vi "Master_Control.vi"(8 "error in (no error)":errorcluster, 10 "FPGA VI Reference In":refnum<k20>) -> (0 "error out":errorcluster, 2 "FPGA VI Reference Out":refnum<k20>)   [LabVIEW 2017]
doc: "The control loop on the cRIO.\nContains the state machine that sets actuations by states. The actuations vary depending on the runtype class used, set from the tab control on the Host Front Panel. Although each variation of the state has similar properties.\nContains an emergency check, watchdog pet/kick, distance approximator.\nThe runtypes are as follows:\nFullRun - pod is configured to perform a vacuum run through the tube at full speed\nSystemsCheck - manual control over all actuations is provided, including a short motor pulse feature\nService - motor is running and manual control over the pod's position is provided\nThe states are as follows:\nIdle - pod is not in motion, and is in a safe state\nReady - all subsystems are actuated and the command to send pod into launch is enabled\nPushing - pod is in motion and accelerating\nCoasting - pod is neither accelerating nor braking\nBraking - pod is braking and coming to a stop\nFault - the emergency check registered a fault and all outputs are disabled\nShutdown - the GlobalStop variable is set to true, stopping all loops running on the cRIO\nBlank - a template for easily creating new states as needed"
uses:
  TypeDef_ControlState.ctl
  RunTypesLibrary/FullRunClass/FullRun.lvclass
  C:/Users/Trevor/Documents/GitHub/SpaceXComp/Master/Control/RunTypesLibrary/RunTypeClass/RunType.lvclass
  TypeDef_DigitalOuts.ctl
  TypeDef_LoopPeriods.ctl
  <vilib>/Platform/TimedLoop/XDataNode/timing_clust.ctl
  <vilib>/Platform/TimedLoop/XDataNode/nitl_modes.ctl
  <vilib>/Platform/TimedLoop/XDataNode/wakeup.ctl
  DAQ/Master_DataControl.ctl
  DAQ/TypeDef_cRIOData.ctl
  IMU/TypeDef_IMUData.ctl
  CAN/TypeDef_BMSData.ctl
  CAN/TypeDef_BMS_Status.ctl
  CAN/MotorController/fixedMotorData.ctl
  CAN/MotorController/MotorStatus.ctl
  RunTypesLibrary/RunTypeList.ctl
  RunTypesLibrary/SystemsCheckClass/SystemsCheck.lvclass
  <vilib>/Platform/TimedLoop/XDataNode/loadnilvce.vi
  <vilib>/platform/TimedLoop/XDataNode/XDataNode.xnode
  RunTypesLibrary/RunTypeClass/RunType.lvclass
  EmergencyCheck/CheckData/CheckData.lvclass
  <vilib>/Platform/TimedLoop/XDataNode/XDNodeRunTimeDep.lvlib
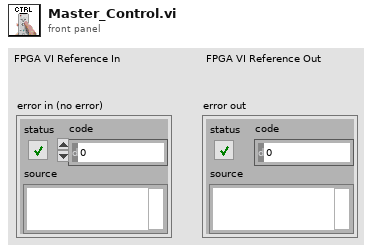
[diagram p1: front panel]
types:
  T1 = typedef "TypeDef_DigitalOuts.ctl" = cluster{"Pod Power":bool, "Dump Valve":bool, "Brakes":bool, "Clamp":bool, "Pump":bool, "Ignition":bool, "DO6":bool, "DO7":bool, "HighSide":bool, "Precharge":bool, "LowSide":bool, "DO3":bool, "DO4":bool, "DO5":bool, "DO62":bool, "DO72":bool}
  T2 = typedef "TypeDef_ControlState.ctl" = enum16{"Systems Check", "Idle", "Ready", "Pushing", "Coast", "Braking", "Fault", "Shutdown", "Service", "Precharge", "Blank"}
  T3 = typedef "TypeDef_LoopPeriods.ctl" = cluster{"Control Period":i64, "DAQ Period":u32, "IMU Period":u32, "CAN Period":i64, "Nav Period":u32}
  T4 = typedef "XDNodeRunTimeDep.lvlib/timing_clust.ctl" = cluster{"Expected End [f-1]":u64, "Actual End [f-1]":u64, "Finished Late? [f-1]":bool, "Expected End [i-1]":u64, "Actual End [i-1]":u64, "Finished Late? [i-1]":bool, "Expected Start [i]":u64, "Actual Start [i]":u64, "Expected Start [f]":u64, "Actual Start [f]":u64, "Source Name":string, "Structure Name":string, "Period":i64, "Deadline":i64, "Offset":i64, "Start":i64, "Priority":i32, "Timeout":i32, "Mode":T5, "Wakeup Reason":T6, "Error":errorcluster, "Source Type":string, "Secondary Source Type":string, "Global End Time":u64, "Global Start Time":u64, "Frame Duration":u64, "Iteration Duration":u64, "Assigned CPU":i32, "I/O Scan Engine Mode":u32}
  T5 = typedef "XDNodeRunTimeDep.lvlib/nitl_modes.ctl" = enum32{"No Change", "Process missed periods, maintain original phase", "Discard missed periods, maintain original phase", "Process missed periods, ignore original phase", "Discard missed periods, ignore original phase"}
  T6 = typedef "XDNodeRunTimeDep.lvlib/wakeup.ctl" = enum32{"Normal", "Aborted", "Asynchronous wakeup", "Timing source error", "Timed loop error", "Timeout"}
  T7 = typedef "RunTypeList.ctl" = enum16{"Full Run", "Systems Check", "Service"}
  T8 = typedef "Master_DataControl.ctl" = cluster{"cRIO Data":T9, "IMU Data":T10, "BMS Data":T11, "Motor Data":T13}
  T9 = typedef "TypeDef_cRIOData.ctl" = cluster{"Time (ms)":dbl, "24V Battery (V)":dbl, "LowV Current (A)":dbl, "Fiducial Sensor (V)":dbl, "PV Pressure (psig)":dbl, "Flow Sensor (V)":dbl, "Temp Fairing (F)":dbl, "Temp Reservoir (F)":dbl, "HallEffect Right (in)":dbl, "HallEffect Left (in)":dbl, "PT Tank (psig)":dbl, "PT Clamp Right (psig)":dbl, "PT Clamp Left (psig)":dbl, "PT Brake (psig)":dbl, "PT Cooling (psig)":dbl, "Displacement (ft)":dbl, "Velocity (ft/s)":dbl}
  T10 = typedef "TypeDef_IMUData.ctl" = cluster{"x acceleration (g)":dbl, "Pressure (psia)":dbl, "Temperature (F)":dbl}
  T11 = typedef "TypeDef_BMSData.ctl" = cluster{"Max Cell Voltage (V)":dbl, "Max Cell ID":dbl, "Min Cell Voltage (V)":dbl, "Min Cell ID":dbl, "State of Charge (%)":dbl, "Average Voltage (V)":dbl, "Voltage Delta (V)":dbl, "Pack Current (A)":dbl, "Pack Voltage (V)":dbl, "Max Resistance (Ohm)":dbl, "Min Resistance (Ohm)":dbl, "Average Resistance (Ohm)":dbl, "Delta Resistance (Ohm)":dbl, "Highest Temperature(F)":dbl, "BmsStatus":T12}
  T12 = typedef "TypeDef_BMS_Status.ctl" = cluster{"isFault":bool, "isolationMonitoring":bool}
  T13 = typedef "fixedMotorData.ctl" = cluster{"Velo (RPM)":dbl, "MotorTemp(F)":dbl, "CtrlTemp(F)":dbl, "DcLinkVolt(V)":dbl, "ErrorCode":dbl, "motorStatus":T14, "isAlive":bool, "motorControllerState":u16}
  T14 = typedef "MotorStatus.ctl" = cluster{"isReady":bool, "isOn":bool, "isOperEn":bool, "isFault":bool, "isVoltEn":bool, "targetReached":bool, "isWarning":bool}
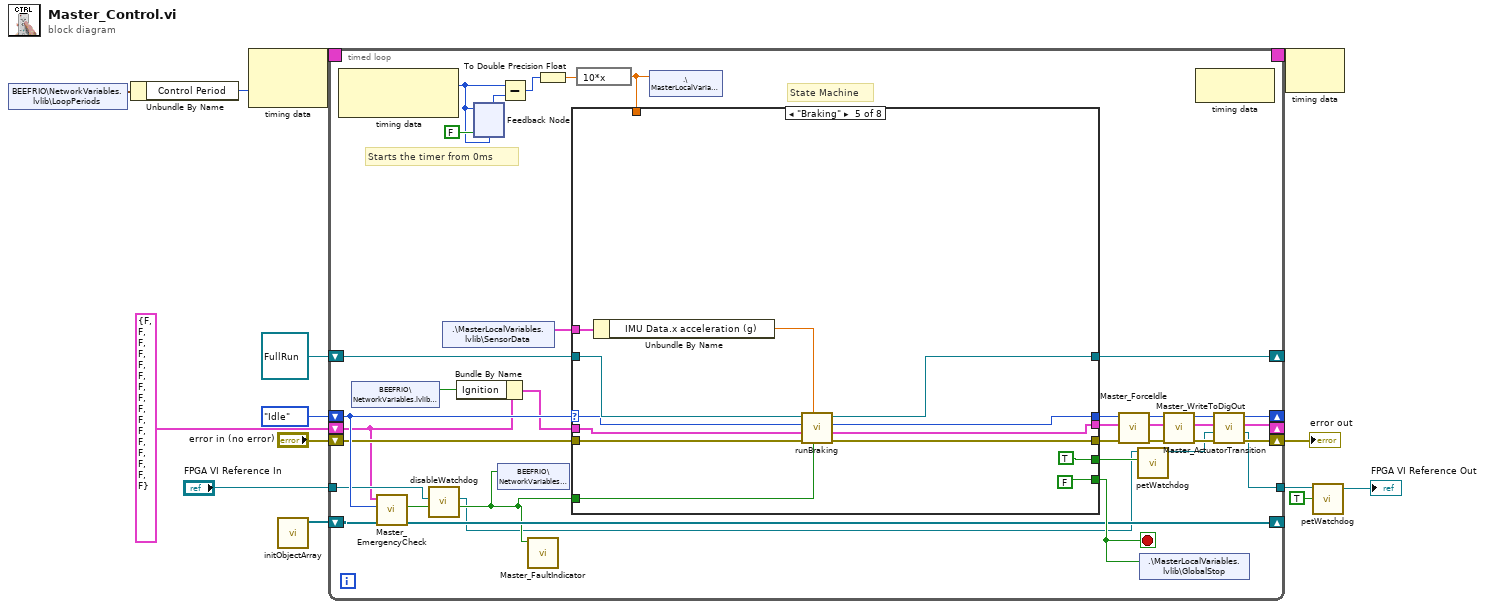
[diagram p0: block diagram]
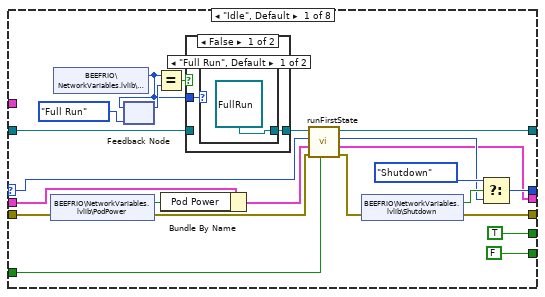
[diagram p2: hidden frame]
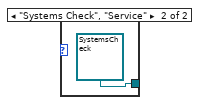
[diagram p3: hidden frame]
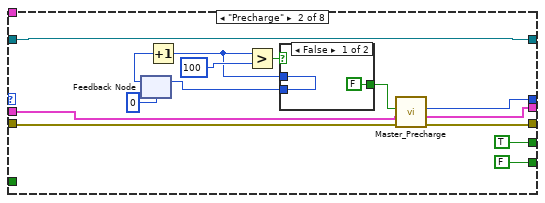
[diagram p5: hidden frame]
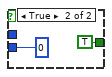
[diagram p6: hidden frame]
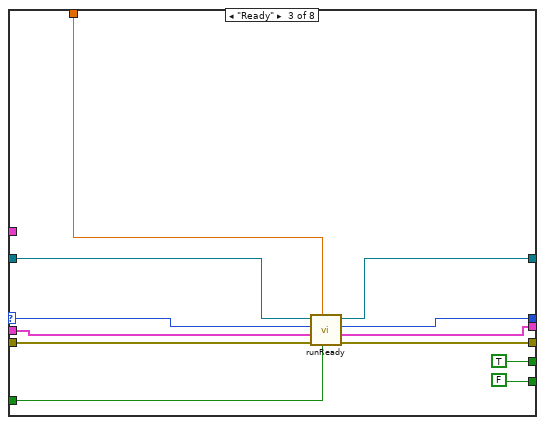
[diagram p7: hidden frame]
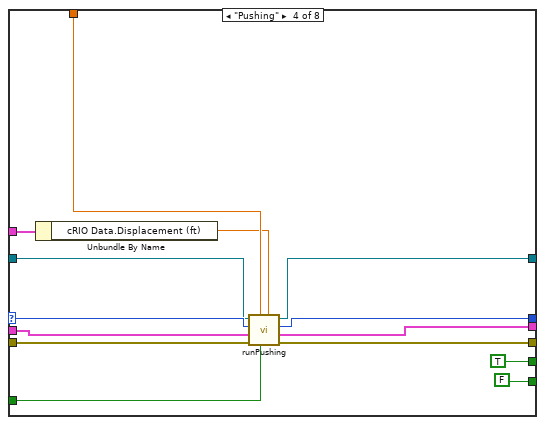
[diagram p8: hidden frame]
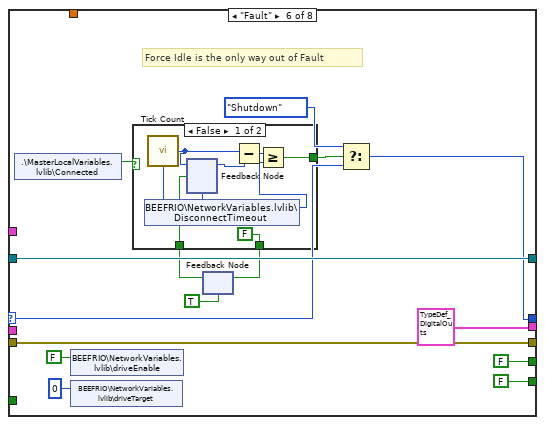
[diagram p9: hidden frame]
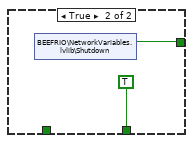
[diagram p10: hidden frame]
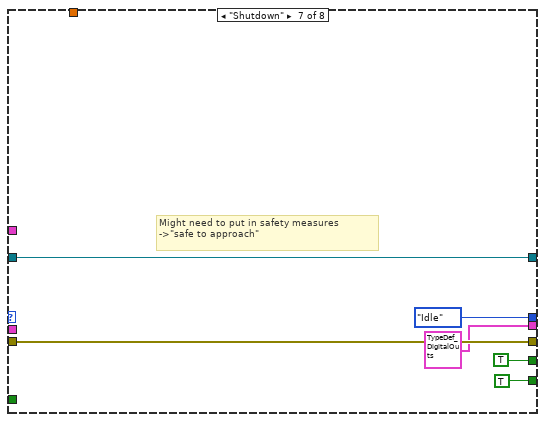
[diagram p11: hidden frame]
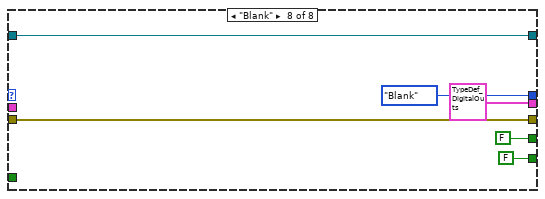
[diagram p12: hidden frame]
diagram:
  n1 = shared-variable "BEEFRIO\\NetworkVariables.lvlib\\LoopPeriods"() -> (w10:T3)  [unwired: 1 in, 1 out]
  n2 = Unbundle By Name(w10) -> ("Control Period"=w9:i64)
  n3 = node-c288(w9) -> (w14:T4)  [unwired: 1 in]
  n4 = call "initObjectArray.vi"() -> ("CheckData out"=w6:refnum<class "CheckData.lvclass">[])  [unwired: 11 in]
  n5 = timed-loop {
    shift-right: [w20] -> _
    shift-left: T1 {"Pod Power"=FALSE, "Dump Valve"=FALSE, "Brakes"=FALSE, "Clamp"=FALSE, "Pump"=FALSE, "Ignition"=FALSE, "DO6"=FALSE, "DO7"=FALSE, "HighSide"=FALSE, "Precharge"=FALSE, "LowSide"=FALSE, "DO3"=FALSE, "DO4"=FALSE, "DO5"=FALSE, "DO62"=FALSE, "DO72"=FALSE} ("Actuators out") -> [w15]
    timing: w14 -> [_]
    timing-out: [_] -> w13
    shift-right: [w44] -> _
    shift-left: TypeDef_ControlState."Idle" -> [w33]
    shift-right: [w37] -> w11
    shift-left: "error in (no error)" -> [w32]
    shift-right: [w39] -> _
    shift-left: refnum<class "FullRun.lvclass"> refnum ("ControlLibrary.lvlib:FullRun.lvclass") -> [w40]
    shift-right: [w29] -> _
    shift-left: w6 -> [w30]
    tunnel: "FPGA VI Reference In" -> [w26]
    tunnel: [w22] -> w5
    stop <- w49 stop-if-true
    # "Starts the timer from 0ms"
    # "State Machine"
    n6 = node-c288() -> (w46:i64)  [unwired: 1 in, 1 out]
    n7 = shared-variable "BEEFRIO\\NetworkVariables.lvlib\\Ignition"() -> (w17:bool)  [unwired: 1 in, 1 out]
    n8 = call "Master_EmergencyCheck.vi"("CheckData in"=w30, "State in"=w33, "Actuators in"=w15) -> ("CheckData out"=w29:refnum<class "CheckData.lvclass">[], "Fault?"=w27:bool)  [unwired: 7 in]
    n9 = call "disableWatchdog.vi"("Fault in"=w27, "FPGA VI Reference In"=w26) -> ("Fault out"=w28:bool, "FPGA VI Reference Out"=w25:refnum<k20>)  [unwired: 8 in]
    n10 = shared-variable ".\\MasterLocalVariables.lvlib\\SensorData"() -> (w18:T8)  [unwired: 1 in, 1 out]
    n11 = Bundle By Name(cluster=w15, "Ignition"=w17) -> (w16:T1)
    n12 = feedback-in #1(w46, FALSE) -> ()
    n13 = feedback #1(w46) -> (w47:i64)
    n14 = shared-variable "BEEFRIO\\NetworkVariables.lvlib\\Fault"(w28) -> ()  [unwired: 1 in, 1 out]
    n15 = Subtract(x=w46, y=w47) -> (x-y=w45:i64)
    n16 = call "Master_FaultIndicator.vi"("Fault in"=w28) -> ()  [unwired: 11 in]
    n17 = To Double Precision Float(number=w45) -> (double precision float=w35:dbl)
    n18 = expression code="10*x"(w35) -> (w34:dbl)
    n19 = case shown="\"Braking\"" w33 {
      selector: w33 -> [w67 _ w108 w122 w131 w144 _ _]
      tunnel: w32 -> [w69 w93 w110 w123 w137 w152 w168 w174]
      tunnel: [w74 w92 w109 w117 w136 w152 w168 w174] -> w24
      tunnel: w28 -> [w63 _ w104 w116 w129 _ _ _]
      tunnel: w18 -> [_ _ _ w113 w133 _ _ _]
      tunnel: [FALSE FALSE FALSE FALSE FALSE FALSE TRUE FALSE] -> w49
      tunnel: w34 -> [_ _ w102 w120 _ _ _ _]
      tunnel: [w73 w91 w107 w118 w130 w143 TypeDef_ControlState."Idle" ("element") TypeDef_ControlState."Blank" ("element")] -> w43
      tunnel: w40 -> [w58 w83 w105 w121 w135 w151 w165 w171]
      tunnel: [w64 w83 w106 w119 w134 w151 w165 w171] -> w39
      tunnel: [TRUE ("RT Safe") TRUE ("RT Safe") TRUE ("RT Safe") TRUE ("RT Safe") TRUE ("RT Safe") FALSE ("RT Safe") TRUE ("RT Safe") FALSE ("RT Safe")] -> w31
      tunnel: w16 -> [w55 w82 w101 w115 w127 _ _ _]
      tunnel: [w53 w81 w100 w114 w126 T1 {"Pod Power"=FALSE, "Dump Valve"=FALSE, "Brakes"=FALSE, "Clamp"=FALSE, "Pump"=FALSE, "Ignition"=FALSE, "DO6"=FALSE, "DO7"=FALSE, "HighSide"=FALSE, "Precharge"=FALSE, "LowSide"=FALSE, "DO3"=FALSE, "DO4"=FALSE, "DO5"=FALSE, "DO62"=FALSE, "DO72"=FALSE} ("Actuators out") T1 {"Pod Power"=FALSE, "Dump Valve"=FALSE, "Brakes"=FALSE, "Clamp"=FALSE, "Pump"=FALSE, "Ignition"=FALSE, "DO6"=FALSE, "DO7"=FALSE, "HighSide"=FALSE, "Precharge"=FALSE, "LowSide"=FALSE, "DO3"=FALSE, "DO4"=FALSE, "DO5"=FALSE, "DO62"=FALSE, "DO72"=FALSE} ("Actuators out") T1 {"Pod Power"=FALSE, "Dump Valve"=FALSE, "Brakes"=FALSE, "Clamp"=FALSE, "Pump"=FALSE, "Ignition"=FALSE, "DO6"=FALSE, "DO7"=FALSE, "HighSide"=FALSE, "Precharge"=FALSE, "LowSide"=FALSE, "DO3"=FALSE, "DO4"=FALSE, "DO5"=FALSE, "DO62"=FALSE, "DO72"=FALSE} ("Actuators out")] -> w19
      frame "Idle", Default {
        n20 = shared-variable "BEEFRIO\\NetworkVariables.lvlib\\PodPower"(error in=w69) -> (w65:bool, error out=w66:errorcluster)
        n21 = shared-variable "BEEFRIO\\NetworkVariables.lvlib\\RunType"() -> (w60:T7)  [unwired: 1 in, 1 out]
        n22 = feedback #2(RunTypeList."Full Run" ("RunType")) -> (w62:T7)
        n23 = feedback-in #2(w60) -> ()
        n24 = Equal?(x=w60, y=w62) -> (x = y?=w61:bool)
        n25 = Bundle By Name(cluster=w55, "Pod Power"=w65) -> (w54:T1)
        n26 = case shown="False" w61 {
          tunnel: w58 -> [_ w80]
          tunnel: w60 -> [w77 _]
          tunnel: [w76 w80] -> w59
          frame False {
            n27 = case shown="\"Full Run\", Default" w77 {
              tunnel: [refnum<class "FullRun.lvclass"> refnum ("ControlLibrary.lvlib:FullRun.lvclass") refnum<class "SystemsCheck.lvclass"> refnum ("ControlLibrary.lvlib:SystemsCheck.lvclass")] -> w76
              frame "Full Run", Default {
              }
              frame "Systems Check", "Service" {
              }
            }
          }
          frame True {
          }
        }
        n28 = call-dynamic "runFirstState.vi"("Fault?"=w63, "error in (no error)"=w66, "Actuators in"=w54, "State in"=w67, "RunType in"=w59) -> ("error out"=w70:errorcluster, "Actuators out"=w53:T1, "State out"=w68:T2, "RunType out"=w64:refnum<class "RunType.lvclass">)  [unwired: 3 in]
        n29 = shared-variable "BEEFRIO\\NetworkVariables.lvlib\\Shutdown"(error in=w70) -> (w72:bool, error out=w74:errorcluster)
        n30 = Select(t=TypeDef_ControlState."Shutdown", s=w72, f=w68) -> (s? t:f=w73:T2)
      }
      frame "Precharge" {
        n31 = feedback #3(u8 0) -> (w89:u8)
        n32 = Increment(x=w89) -> (x+1=w85:u8)
        n33 = Greater?(x=w85, y=u8 100) -> (0:w87:bool)
        n34 = case shown="False" w87 {
          tunnel: [FALSE TRUE] -> w86
          tunnel: w85 -> [w96 _]
          tunnel: [w96 u8 0] -> w84
          frame False {
          }
          frame True {
          }
        }
        n35 = feedback-in #3(w84) -> ()
        n36 = call "Master_Precharge.vi"("error in (no error)"=w93, "Actuators in"=w82, "Time complete?"=w86) -> ("error out"=w92:errorcluster, "Actuators out"=w81:T1, "State out"=w91:T2)  [unwired: 6 in]
      }
      frame "Ready" {
        n37 = call-dynamic "runReady.vi"("Fault?"=w104, "Time in"=w102, "error in (no error)"=w110, "Actuators in"=w101, "State in"=w108, "RunType in"=w105) -> ("error out"=w109:errorcluster, "Actuators out"=w100:T1, "State out"=w107:T2, "RunType out"=w106:refnum<class "RunType.lvclass">)  [unwired: 1 in, 1 out]
      }
      frame "Pushing" {
        n38 = Unbundle By Name(w113) -> ("cRIO Data.Displacement (ft)"=w112:dbl)
        n39 = call-dynamic "runPushing.vi"("Distance"=w112, "Fault?"=w116, "Time"=w120, "error in (no error)"=w123, "Actuators in"=w115, "State in"=w122, "RunType in"=w121) -> ("error out"=w117:errorcluster, "Actuators out"=w114:T1, "State out"=w118:T2, "RunType out"=w119:refnum<class "RunType.lvclass">)  [unwired: 1 in]
      }
      frame "Braking" {
        n40 = Unbundle By Name(w133) -> ("IMU Data.x acceleration (g)"=w132:dbl)
        n41 = call-dynamic "runBraking.vi"("Fault?"=w129, "x acceleration"=w132, "error in (no error)"=w137, "Actuators in"=w127, "State in"=w131, "RunType in"=w135) -> ("error out"=w136:errorcluster, "Actuators out"=w126:T1, "State out"=w130:T2, "RunType out"=w134:refnum<class "RunType.lvclass">)  [unwired: 2 in]
      }
      frame "Fault" {
        # "Force Idle is the only way out of Fault"
        n42 = shared-variable ".\\MasterLocalVariables.lvlib\\Connected"() -> (w139:bool)  [unwired: 1 in, 1 out]
        n43 = shared-variable "BEEFRIO\\NetworkVariables.lvlib\\driveEnable"(FALSE ("driveEnable")) -> ()  [unwired: 1 in, 1 out]
        n44 = shared-variable "BEEFRIO\\NetworkVariables.lvlib\\driveTarget"(i16 0 ("driveTarget")) -> ()  [unwired: 1 in, 1 out]
        n45 = feedback #4(TRUE) -> (w140:bool)
        n46 = case shown="False" w139 {
          tunnel: [w157 w161] -> w145
          tunnel: [FALSE TRUE] -> w141
          tunnel: w140 -> [w155 _]
          frame False {
            n47 = shared-variable "BEEFRIO\\NetworkVariables.lvlib\\DisconnectTimeout"() -> (w154:u32)  [unwired: 1 in, 1 out]
            n48 = call "Tick Count"() -> ("Tick Count(mSec)"=w159:u32)
            n49 = feedback #5(w159) -> (w160:u32)
            n50 = feedback-in #5(w159, w155) -> ()
            n51 = Subtract(x=w159, y=w160) -> (x-y=w158:u32)
            n52 = Greater Or Equal?(x=w158, y=w154) -> (x >= y?=w157:bool)
          }
          frame True {
            n53 = shared-variable "BEEFRIO\\NetworkVariables.lvlib\\Shutdown"() -> (w161:bool)  [unwired: 1 in, 1 out]
          }
        }
        n54 = feedback-in #4(w141) -> ()
        n55 = Select(t=TypeDef_ControlState."Shutdown", s=w145, f=w144) -> (s? t:f=w143:T2)
      }
      frame "Shutdown" {
        # "Might need to put in safety measures\n->\"safe to approach\""
      }
      frame "Blank" {
      }
    }
    n56 = shared-variable ".\\MasterLocalVariables.lvlib\\Time"(w34) -> ()  [unwired: 1 in, 1 out]
    n57 = call "Master_ForceIdle.vi"("error in"=w24, "Actuators in"=w19, "State In"=w43) -> ("error out"=w41:errorcluster, "Actuators out"=w36:T1, "State Out"=w42:T2)  [unwired: 6 in]
    n58 = call "petWatchdog.vi"("RT Safe"=w31, "FPGA VI Reference In"=w25) -> ("FPGA VI Reference Out"=w23:refnum<k20>)  [unwired: 9 in]
    n59 = shared-variable ".\\MasterLocalVariables.lvlib\\GlobalStop"(w49) -> ()  [unwired: 1 in, 1 out]
    n60 = call "Master_ActuatorTransition.vi"("error in (no error)"=w41, "Actuators in"=w36, "element in"=w42) -> ("error out"=w38:errorcluster, "Actuators out"=w21:T1, "element out"=w44:T2)  [unwired: 6 in]
    n61 = node-c288() -> ()  [unwired: 1 in, 1 out]
    n62 = call "Master_WriteToDigOut.vi"("error in"=w38, "FPGA VI Reference In"=w23, "Actuators in"=w21) -> ("error out"=w37:errorcluster, "FPGA VI Reference Out"=w22:refnum<k20>, "Actuators out"=w20:T1)  [unwired: 6 in]
  }
  "error out" <- w11
  n63 = node-c288(w13) -> ()  [unwired: 1 out]
  n64 = call "petWatchdog.vi"("RT Safe"=TRUE, "FPGA VI Reference In"=w5) -> ("FPGA VI Reference Out"=→"FPGA VI Reference Out":refnum<k20>)  [unwired: 9 in]
